vi "Actor Core.vi"(8 "error in":errorcluster, 11 "ModelPublishesDblX in":refnum<class "ModelPublishesDblX.lvclass">) -> (0 "error out":errorcluster, 3 "Actor out":refnum<class "Actor.lvclass">)   [LabVIEW 2020, in "ModelPublishesDblX.lvclass"]
doc: "(<B>Filename</B>: Actor Framework.lvlib:Actor.lvclass:Actor Core.vi)\n\nReceives messages to the actor, reacts to them, and initiates any error handling that may shut the actor down.\n\nDescendant classes may override this VI to append parallel tasks for the actor to complete while it handles messages. Overrides use the Call Parent Method node."
uses:
  ModelPublishesDblX.lvclass
  <vilib>/ActorFramework/Actor/Actor.lvclass
  modules/mva-core/Source/IObserver/IObserver/IObserver.lvclass/IObserver.ctl
  modules/mva-core/Source/IModel/IModel/IModel.lvclass/IModel.ctl
  modules/mva-core/Source/IMediator/PublishRequest/PublishRequest.lvclass/PublishRequest.ctl
  modules/mva-core/Source/IMediator/IMediator Messages/Publish Msg/Publish Msg.lvclass/Publish Msg.ctl
  modules/composed-af-messages/Source/RoundTripMessage/RoundTripMessage.lvclass/RoundTripMessage.ctl
  <vilib>/ActorFramework/Message Enqueuer/Message Enqueuer.lvclass/Message Enqueuer.ctl
  modules/mva-core/Source/IMediator/IMediator Messages/Publish Msg/Send Pre-Addressed Publish.vi
  modules/mva-core/Source/IObserver/IObserver/Read Unique ID.vi
  modules/mva-core/Source/IMediator/PublishRequest/Pack Publish Request.vi
  modules/composed-af-messages/Source/RoundTripMessage/Return Round-Trip Message.vi
  <vilib>/ActorFramework/Message Enqueuer/Enqueue.vi
  modules/mva-core/Source/IModel/IModel/IModel.lvclass
  modules/mva-core/Source/IMediator/IMediator Messages/Publish Msg/Publish Msg.lvclass
  modules/composed-af-messages/Source/RoundTripMessage/RoundTripMessage.lvclass
  C:/Program Files/National Instruments/LabVIEW 2020/vi.lib/ActorFramework/Message/Message.lvclass
  <vilib>/Utility/error.llb/Error Cluster From Error Code.vi
  <vilib>/ActorFramework/Message Priority Queue/Priority Enqueue.vi
  modules/mva-core/Source/IMediator/PublishRequest/PublishRequest.lvclass
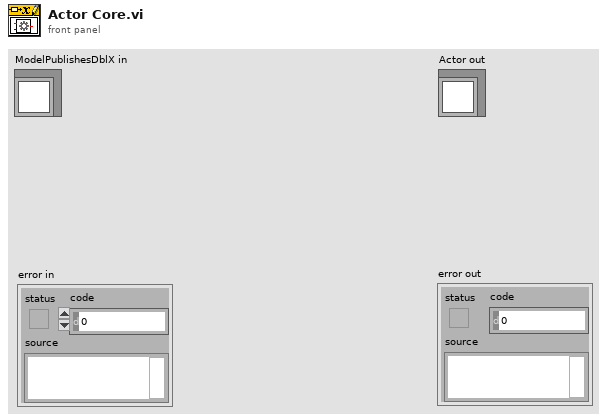
[diagram p1: front panel]
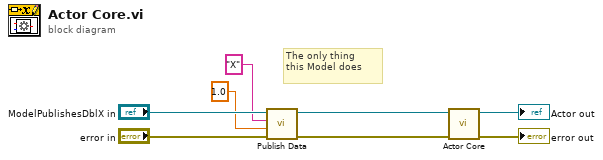
[diagram p0: block diagram]
diagram:
  # "The only thing\nthis Model does"
  n1 = call "Publish Data.vi"("error in (no error)"="error in", "Data to Publish"=1.0, "Datum Name"="X", "IModel in"="ModelPublishesDblX in") -> ("error out"=w5:errorcluster, "IModel out"=w3:refnum<class "ModelPublishesDblX.lvclass">)  [unwired: 6 in]
  n2 = call-parent "Actor Core.vi"("error in"=w5, "Actor in"=w3) -> ("error out"=→"error out":errorcluster, "Actor out"=→"Actor out":refnum<class "Actor.lvclass">)  [unwired: 8 in]
